vi "Update Enum Setter.vi"(7 "RPC Message Name":string, 8 "error in (no error)":errorcluster, 10 "Message Getter in":refnum<vi>, 11 "RPC Messages Folder (ProjectItem) in":refnum<vi>) -> (0 "error out":errorcluster, 2 "Message Getter out":refnum<vi>, 3 "RPC Messages Folder (ProjectItem) out":refnum<vi>)   [LabVIEW 2019, in "gRPC Template Creation Utility.lvlib"]
uses:
  gRPC Template Creation Utility.lvlib
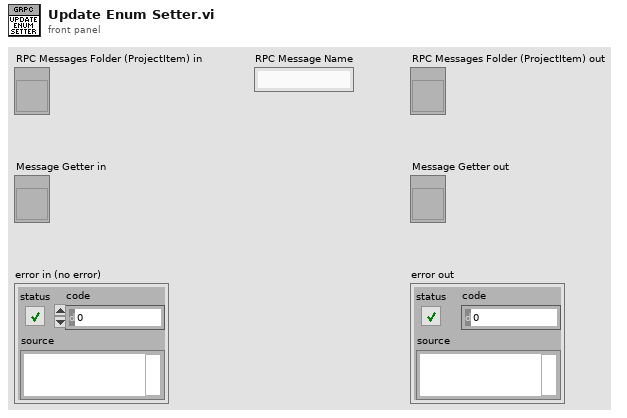
[diagram p1: front panel]
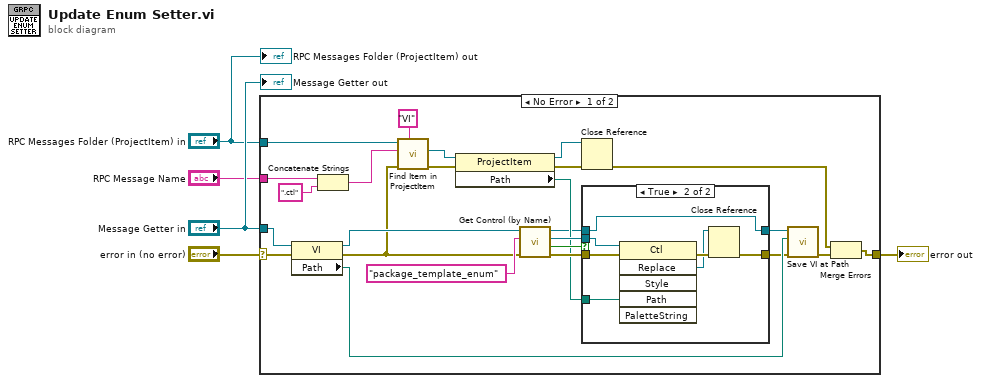
[diagram p0: block diagram]
diagram:
  n1 = case shown="No Error" "error in (no error)" {
    selector: "error in (no error)" -> [w12 w40]
    tunnel: "Message Getter in" -> [w29 _]
    tunnel: [w28 w40] -> w4
    tunnel: "RPC Message Name" -> [w19 _]
    tunnel: "RPC Messages Folder (ProjectItem) in" -> [w17 _]
    frame No Error {
      n2 = property class="VI"(reference=w29, error in=w12) -> (reference out=w13:refnum<vi>, error out=w8:errorcluster, "Path"=w30:path)
      n3 = Concatenate Strings(w19, ".ctl" ("string")) -> (w21:string)
      n4 = call "Find Item in ProjectItem.vi"("Item Type"="VI", "error in (no error)"=w8, "Name"=w21, "ProjectItem in"=w17) -> ("error out"=w23:errorcluster, "Item Refnum out"=w22:refnum<vi>)  [unwired: 4 in, 2 out]
      n5 = property class="ProjectItem"(reference=w22, error in=w23) -> (reference out=w24:refnum<vi>, error out=w25:errorcluster, "Path"=w10:path)
      n6 = call "Get Control (by Name).vi"("error in (no error)"=w8, "Control Label"="package_template_enum" ("name/order"), "Owner VI in"=w13) -> ("error out"=w15:errorcluster, "Found ?"=w16:bool, "Control Refnum"=w14:refnum<vi>, "Owner VI out"=w7:refnum<vi>)  [unwired: 5 in]
      n7 = Close Reference(reference=w24, error in (no error)=w25) -> (error out=w27:errorcluster)
      n8 = case shown="True" w16 {
        tunnel: [w32 w39] -> w9
        tunnel: w14 -> [_ w36]
        tunnel: w15 -> [w32 w35]
        tunnel: w10 -> [_ w34]
        tunnel: w7 -> [w31 w33]
        tunnel: [w31 w33] -> w6
        frame False {
        }
        frame True {
          n9 = invoke class="Ctl" method="Replace"(reference=w36, error in=w35, "Path"=w34) -> (error out=w38:errorcluster, "Replace"=w37:refnum<vi>)  [unwired: 3 in, 4 out]
          n10 = Close Reference(reference=w37, error in (no error)=w38) -> (error out=w39:errorcluster)
        }
      }
      n11 = call "Save VI at Path.vi"("error in (no error)"=w9, "Path"=w30, "VI in"=w6) -> ("error out"=w26:errorcluster)  [unwired: 6 in, 2 out]
      n12 = Merge Errors(w27, w26) -> (w28:errorcluster)
    }
    frame Error {
    }
  }
  "error out" <- w4
  "RPC Messages Folder (ProjectItem) out" <- "RPC Messages Folder (ProjectItem) in"
  "Message Getter out" <- "Message Getter in"
